vi "Test_iLOGAcquisition.vi"() -> ()   [LabVIEW 2019]
uses:
  ByteQXAPIBase/iLOGAcquisition/Acquisitions.ctl
  ByteQXAPIBase/ByteQXAPIBase.lvclass
panel:
  in  "acquisitions":T1[](array[typedef]) {"timestamp" format="%<%x %.3X>T"}
  out "test passed?":bool
  out "error out":errorcluster
  in  "asset code":string
  in  "Auth token":string
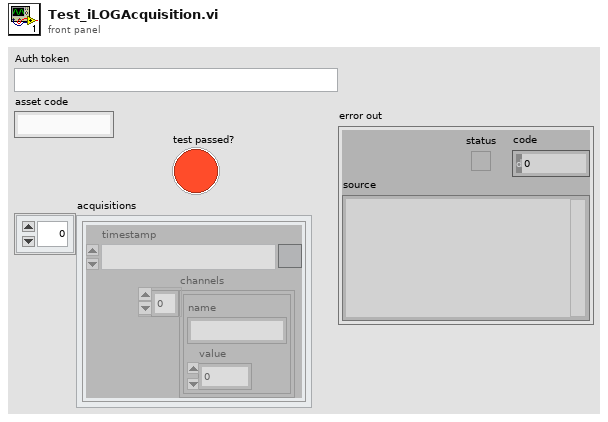
[diagram p1: front panel]
types:
  T1 = typedef "ByteQXWebAPI.lvlib/ByteQXAPIBase.lvclass/Acquisitions.ctl" = cluster{"timestamp":timestamp, "channels":cluster{"name":string, "value":dbl}[]}
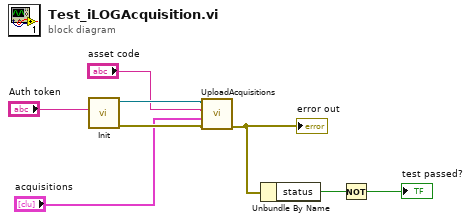
[diagram p0: block diagram]
diagram:
  n1 = call "Init.vi"("Auth token"="Auth token") -> ("error out"=w5:errorcluster, "ByteQXAPIBase out"=w4:refnum<class "ByteQXAPIBase.lvclass">)  [unwired: 9 in]
  n2 = call-dynamic "UploadAcquisitions.vi"("error in (no error)"=w5, "acquisitions"="acquisitions", "asset code"="asset code", "ByteQXAPIBase in"=w4) -> ("error out"=w2:errorcluster)  [unwired: 6 in, 1 out]
  "error out" <- w2
  n3 = Unbundle By Name(w2) -> ("status"=w7:bool)
  n4 = Not(x=w7) -> (.not. x?=→"test passed?":bool)
